vi "get part numbers.vi"() -> (2 "Part numbers":string[](array[string]), 3 "First part":string)   [LabVIEW 2021]
panel:
  out "error out":errorcluster
  in  "error in":errorcluster
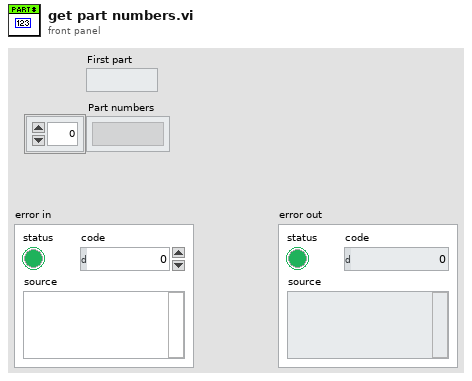
[diagram p1: front panel]
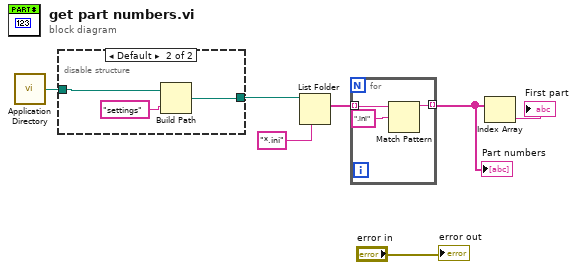
[diagram p0: block diagram]
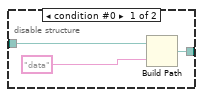
[diagram p2: hidden frame]
diagram:
  n1 = call <vilib>:"Application Directory.vi"() -> ("Application Directory"=w2:path)
  n2 = disable-structure shown="Default" {
    disable-tunnel: [w8 w11] -> w1
    disable-tunnel: w2 -> [w9 w12]
    frame condition #0 {
      n3 = Build Path(base path=w9, name or relative path="data") -> (appended path=w8:path)
    }
    frame condition #1 (active) {
      n4 = Build Path(base path=w12, name or relative path="settings") -> (appended path=w11:path)
    }
  }
  n5 = List Folder(path=w1, pattern="*.ini") -> (filenames=w6:string[])  [unwired: 2 in, 3 out]
  n6 = for {
    tunnel: w6 -> [w15] mode=indexing
    tunnel: [w14] -> w5 mode=indexing
    n7 = Match Pattern(string=w15, regular expression=".ini") -> (before substring=w14:string)  [unwired: 1 in, 3 out]
  }
  "Part numbers" <- w5
  n8 = Index Array(array=w5) -> (element=→"First part":string)  [unwired: 1 in]
  "error out" <- "error in"
